vi "Initialize.vi"(5 "ballast [bytes]":i32, 7 "shift [characters]":u8, 11 "letter":string) -> (3 "Letter out":refnum<class "Letter.lvclass">)   [LabVIEW 2015, in "Letter.lvclass"]
uses:
  Letter.lvclass
  Letter.lvclass/Letter.ctl
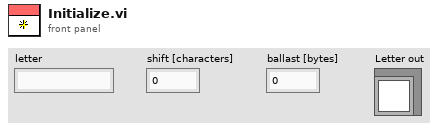
[diagram p1: front panel]
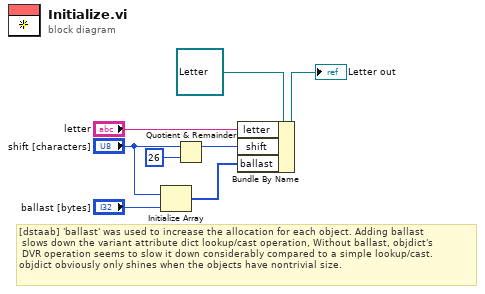
[diagram p0: block diagram]
diagram:
  # "[dstaab] 'ballast' was used to increase the allocation for each object. Adding ballast\n slows down the variant attribute dict lookup/cast operation, Without ballast, objdict's\n DVR operation seems to slow it down considerably compared to a simple lookup/cast.\nobjdict obviously only shines when the objects have nontrivial size."
  n1 = Initialize Array("shift [characters]", "ballast [bytes]") -> (w1:u8[])
  n2 = Quotient & Remainder(x="shift [characters]", y=u8 26) -> (x-y*floor(x/y)=w5:u8)  [unwired: 1 out]
  n3 = Bundle By Name(cluster=refnum<class "Letter.lvclass"> refnum, "letter"="letter", "shift"=w5, "ballast"=w1) -> (→"Letter out":refnum<class "Letter.lvclass">)
